vi "Finder_Max_Min_MB.vi"(2 "Señal\nAcelerómetro":sgl[](array[numeric])) -> (6 "Max, Mín":sgl[](array[numeric]), 9 "Posiciones":i32[](array[numeric]))   [LabVIEW 2015]
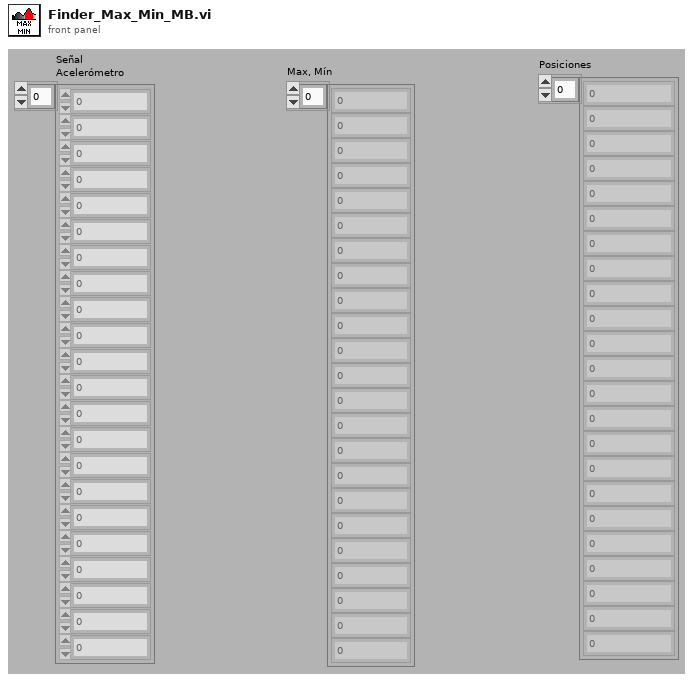
[diagram p1: front panel]
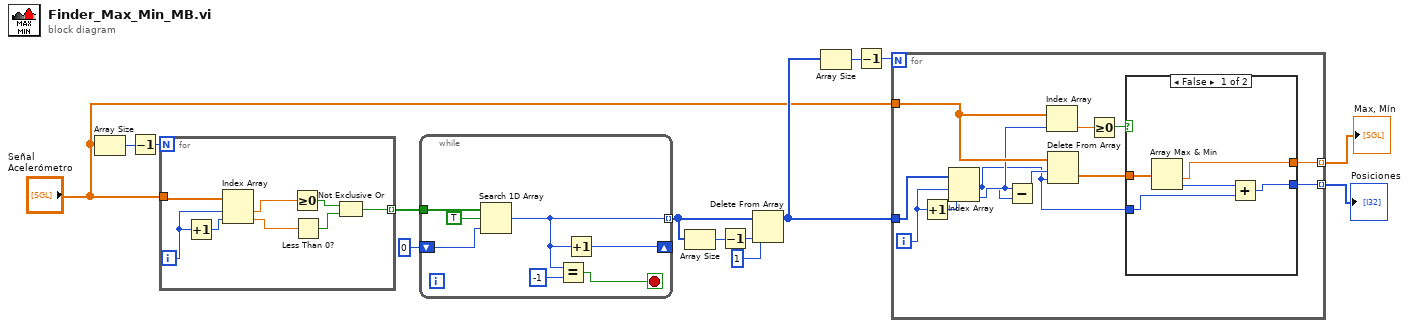
[diagram p0: block diagram]
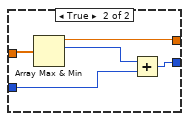
[diagram p2: hidden frame]
diagram:
  n1 = Array Size(array="Señal\nAcelerómetro") -> (size(s)=w14:i32)
  n2 = Decrement(x=w14) -> (x-1=w13:i32)
  n3 = for {
    N: w13 -> [_]
    tunnel: "Señal\nAcelerómetro" -> [w22]
    tunnel: [w15] -> w12 mode=indexing
    i -> [w21]
    n4 = Increment(x=w21) -> (x+1=w20:i32)
    n5 = Index Array(array=w22, index #1=w21, index #2=w20) -> (element #1=w19:sgl, element #2=w18:sgl)
    n6 = Greater Or Equal To 0?(x=w19) -> (x >= 0?=w17:bool)
    n7 = Less Than 0?(x=w18) -> (x < 0?=w16:bool)
    n8 = Not Exclusive Or(1:w16, 2:w17) -> (0:w15:bool)
  }
  n9 = while {
    tunnel: w12 -> [w29]
    tunnel: [w25] -> w10 mode=indexing
    shift-right: [w26] -> _
    shift-left: 0 ("index of element") -> [w27]
    stop <- w23 stop-if-true
    n10 = Search 1D Array(1D array=w29, element=TRUE, start index (0)=w27) -> (index of element=w25:i32)
    n11 = Equal?(x=w25, y=-1) -> (x = y?=w23:bool)
    n12 = Increment(x=w25) -> (x+1=w26:i32)
  }
  n13 = Array Size(array=w10) -> (size(s)=w9:i32)
  n14 = Decrement(x=w9) -> (x-1=w8:i32)
  n15 = Delete From Array(array=w10, length=1, index=w8) -> (array with subset deleted=w4:i32[])  [unwired: 1 out]
  n16 = Array Size(array=w4) -> (size(s)=w6:i32)
  n17 = Decrement(x=w6) -> (x-1=w5:i32)
  n18 = for {
    N: w5 -> [_]
    tunnel: w4 -> [w41]
    tunnel: "Señal\nAcelerómetro" -> [w39]
    tunnel: [w35] -> w3 mode=indexing
    tunnel: [w34] -> w2 mode=indexing
    i -> [w32]
    n19 = Increment(x=w32) -> (x+1=w31:i32)
    n20 = Index Array(array=w41, index #1=w32, index #2=w31) -> (element #1=w30:i32, element #2=w33:i32)
    n21 = Subtract(x=w33, y=w30) -> (x-y=w40:i32)
    n22 = Index Array(array=w39, index=w33) -> (element=w38:sgl)
    n23 = Delete From Array(array=w39, length=w40, index=w30) -> (deleted portion=w36:sgl[])  [unwired: 1 out]
    n24 = Greater Or Equal To 0?(x=w38) -> (x >= 0?=w37:bool)
    n25 = case shown="False" w37 {
      tunnel: w36 -> [w46 w51]
      tunnel: [w45 w50] -> w35
      tunnel: [w42 w47] -> w34
      tunnel: w30 -> [w44 w48]
      frame False {
        n26 = Array Max & Min(array=w46) -> (min value=w45:sgl, min index (indices)=w43:i32)  [unwired: 2 out]
        n27 = Add(x=w43, y=w44) -> (x+y=w42:i32)
      }
      frame True {
        n28 = Array Max & Min(array=w51) -> (max value=w50:sgl, max index (indices)=w49:i32)  [unwired: 2 out]
        n29 = Add(x=w49, y=w48) -> (x+y=w47:i32)
      }
    }
  }
  "Max, Mín" <- w3
  "Posiciones" <- w2
